vi "calib main.vi"() -> ()   [LabVIEW 2019]
uses:
  <vilib>/Utility/miscctls.llb/LVRowAndColumnTypeDef.ctl
  software/database.lvlib
  <vilib>/addons/Multicore Analysis and Sparse Matrix/Linear Algebra/NI_MASM_BasicLinAlg.lvlib
  <vilib>/Analysis/Matrix/NI_Matrix.lvlib
  software/detectedPellet.lvlib
  <vilib>/Analysis/Matrix/Numeric/Conversions/Array To Matrix - RA2.vi
  <vilib>/addons/Multicore Analysis and Sparse Matrix/Linear Algebra/_linalg/Solve Least Squares Problems (DBL).vi
panel:
  out "array":string[][](array[string])
  out "element":string
  out "Row":i32
  out "subarray":string[](array[string])
  out "Processing Table":string[][](table)
  in  "Numeric":i32=26
  in  "Stop (F)":bool
  out "Image Out":T1(plugin-control)
  out "output array":dbl[][](array[numeric])
  out "Error out":errorcluster
  in  "save_DB":bool
  out "Image":T1(plugin-control)
  in  "module path 2":path
  in  "process":bool
  out "Error out 5":errorcluster
  out "input array":dbl[][](array[numeric])
  out "known vector":dbl[](array[numeric])
  out "return value":dbl[](array[numeric])
  out "error out":errorcluster
  in  "module path":path
  out "Image Out 2":T1(plugin-control)
  out "Solution Vector":dbl[](array[numeric])
  in  "calculate":bool
  in  "capture":bool
  in  "snap number":u16(ring) items=["first", "second", "third"]
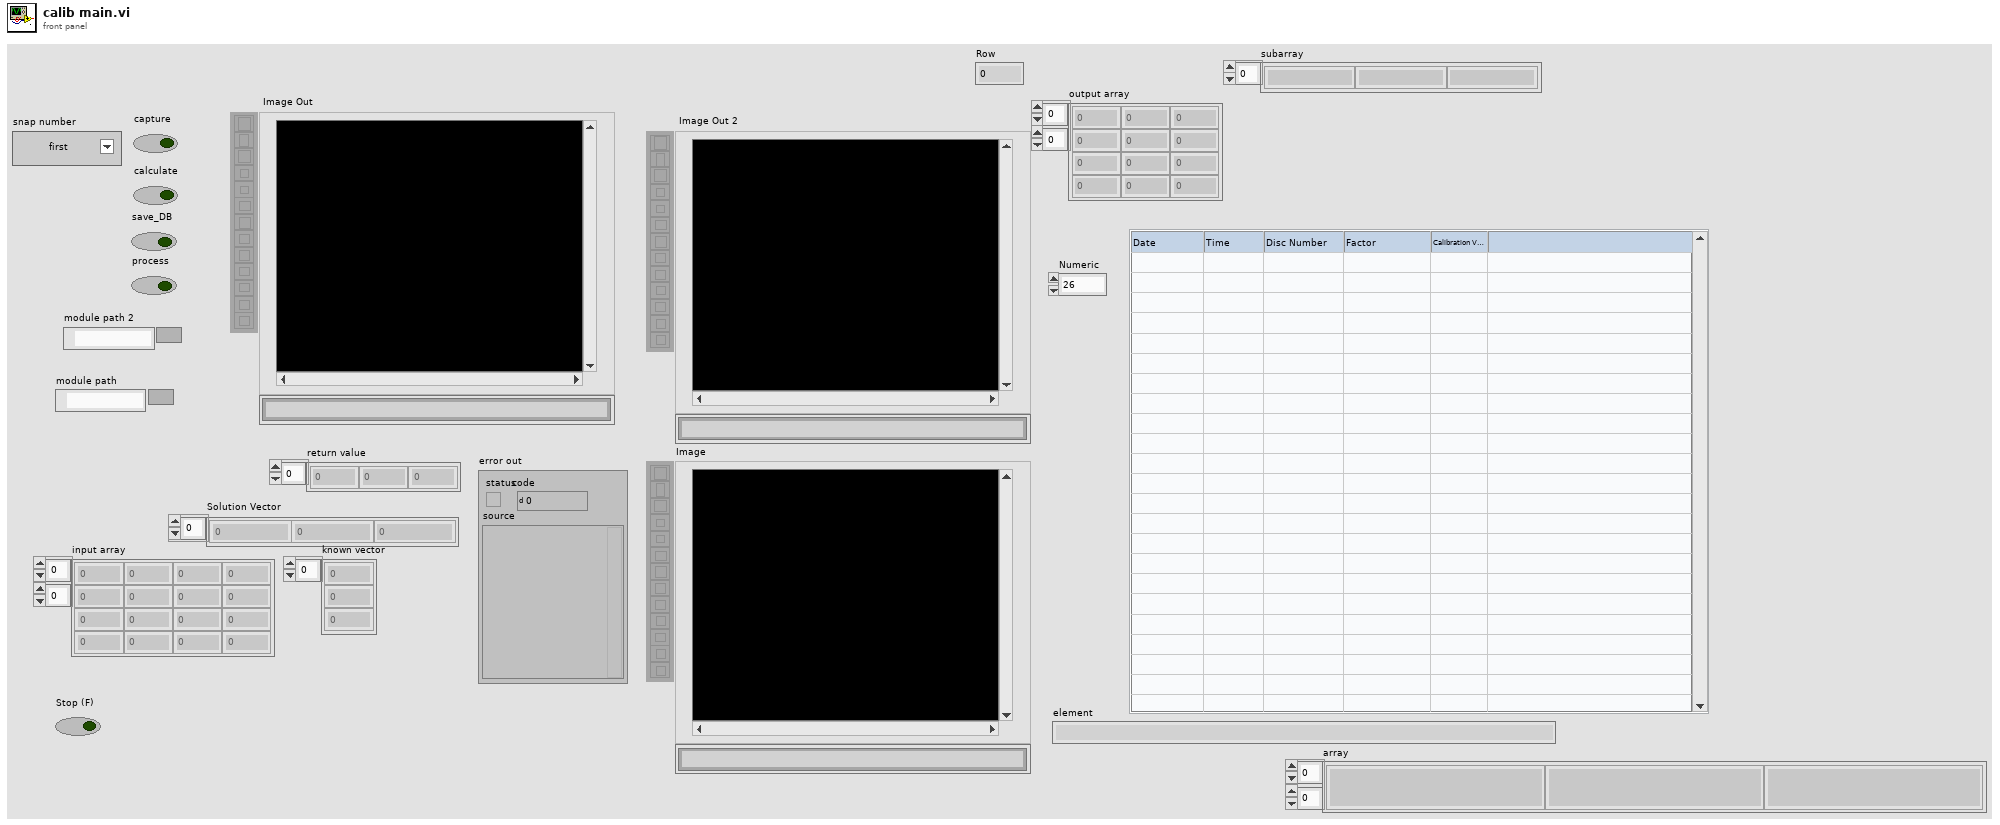
[diagram p1: front panel]
types:
  T1 = typedef "IMAQ Image.ctl" = refnum<image>
  T2 = typedef "Image Type" = u32
  T3 = typedef "LVRowAndColumnTypeDef.ctl" = cluster{"Row":i32, "Column":i32}
  T4 = cluster{"date/time string":string, "date/time string":string, "Numeric":i32, "spreadsheet string":string, "spreadsheet string":string}
  T5 = typedef "NI_Matrix.lvlib/RealMatrix.ctl" = dbl[][]
  T6 = cluster{"date/time string":string, "date/time string":string, "Numeric":dbl, "Numeric":dbl, "Numeric":dbl}
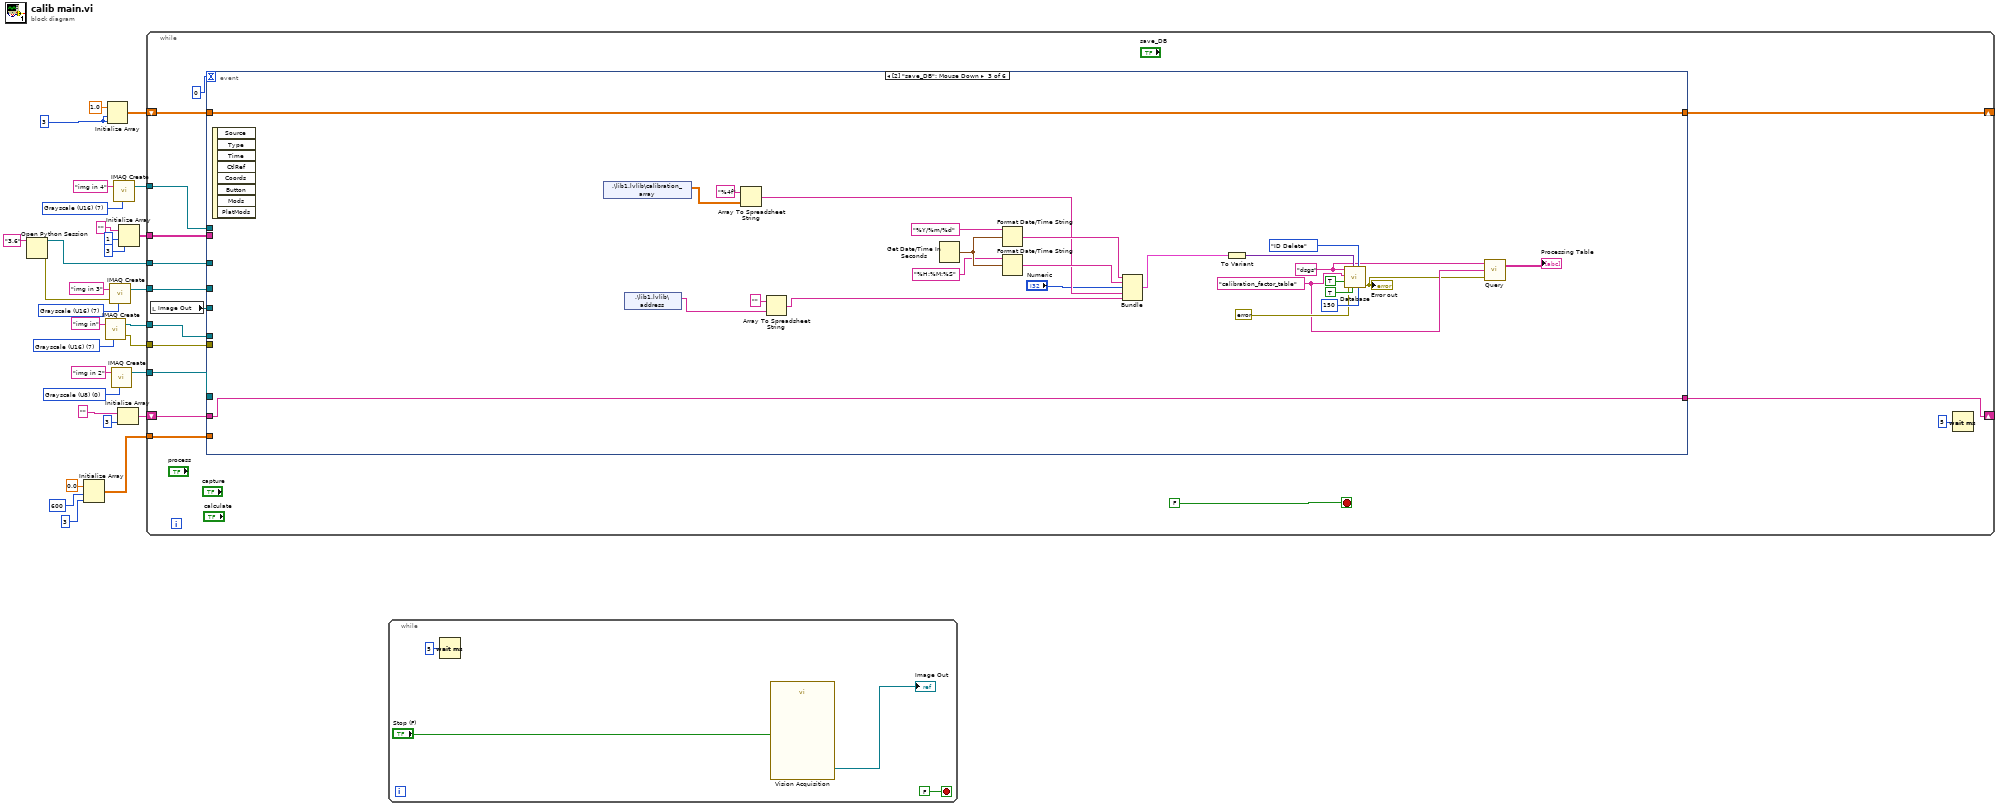
[diagram p0: block diagram]
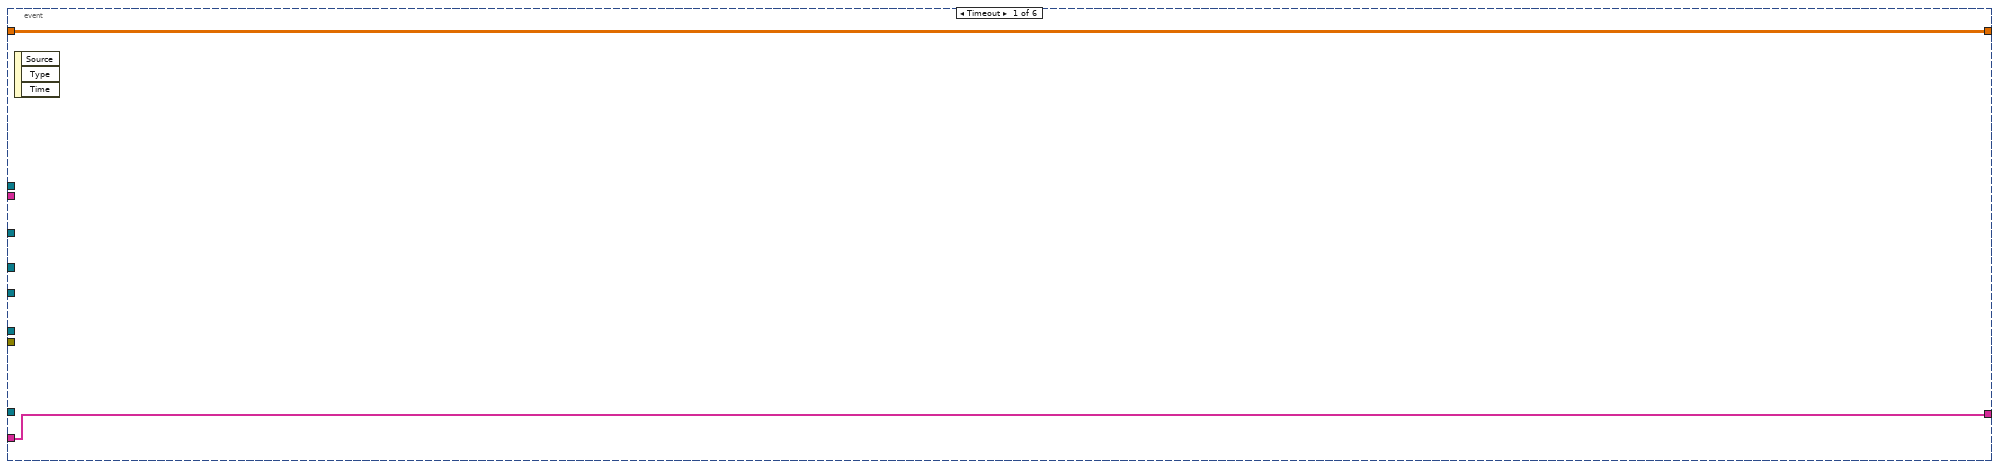
[diagram p2: hidden frame]
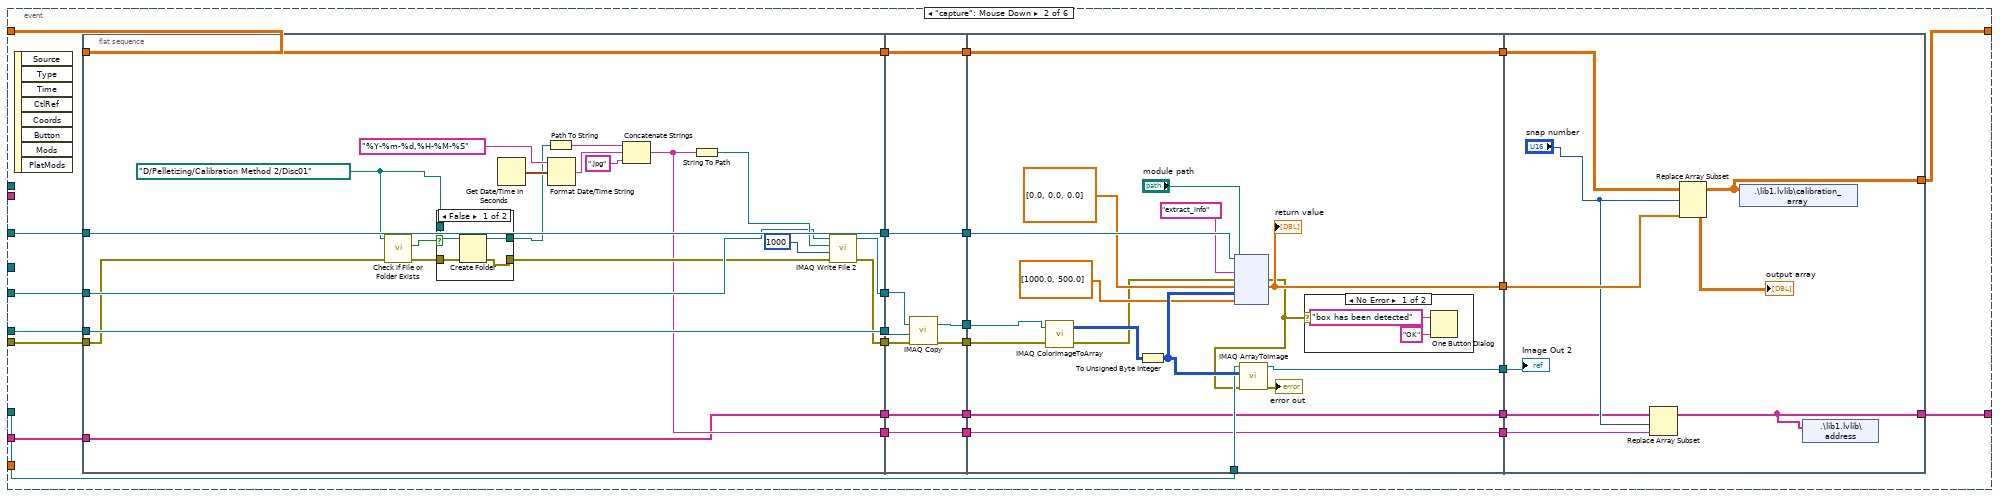
[diagram p3: hidden frame]
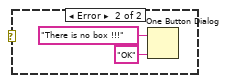
[diagram p5: hidden frame]
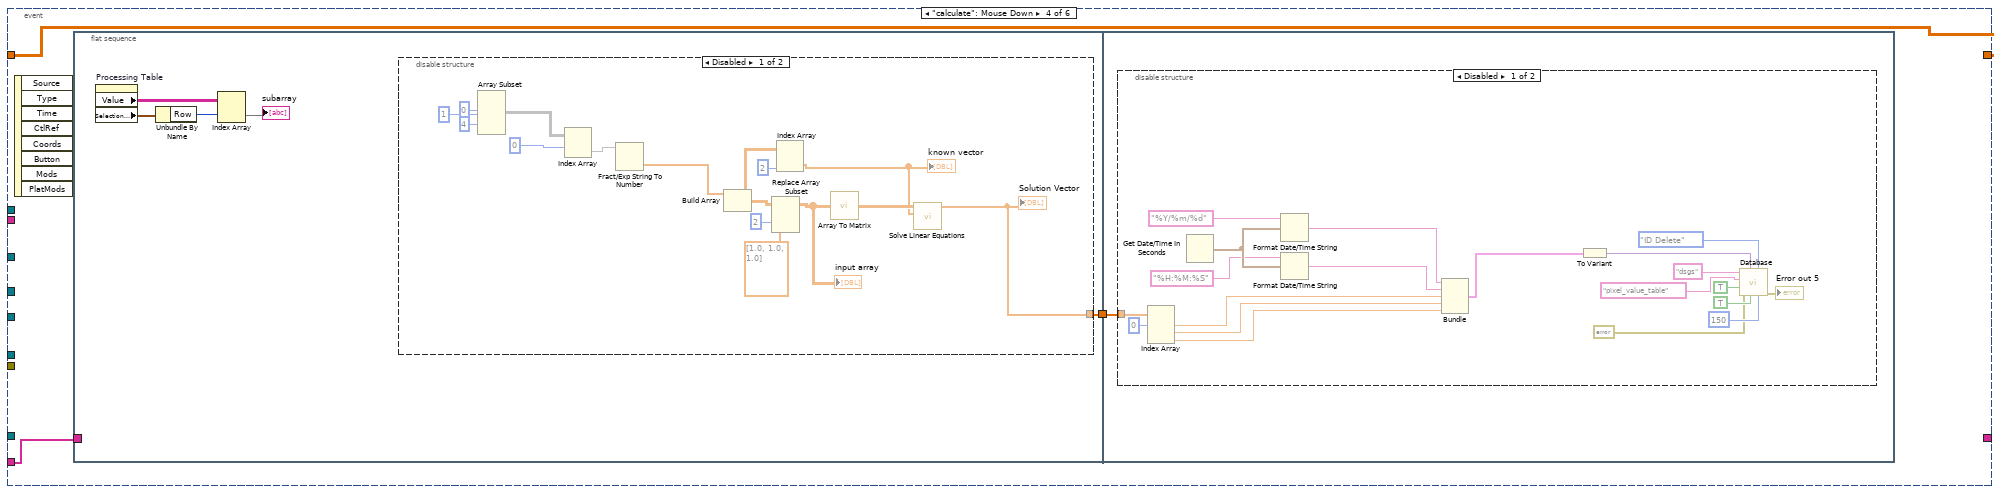
[diagram p6: hidden frame]
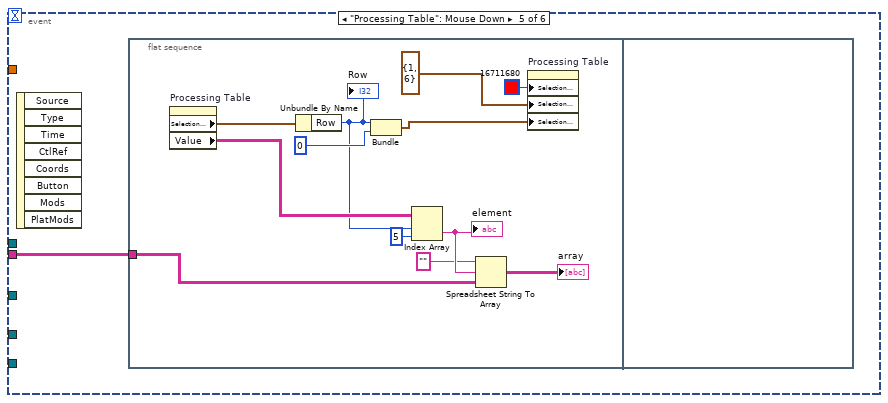
[diagram p9: hidden frame]
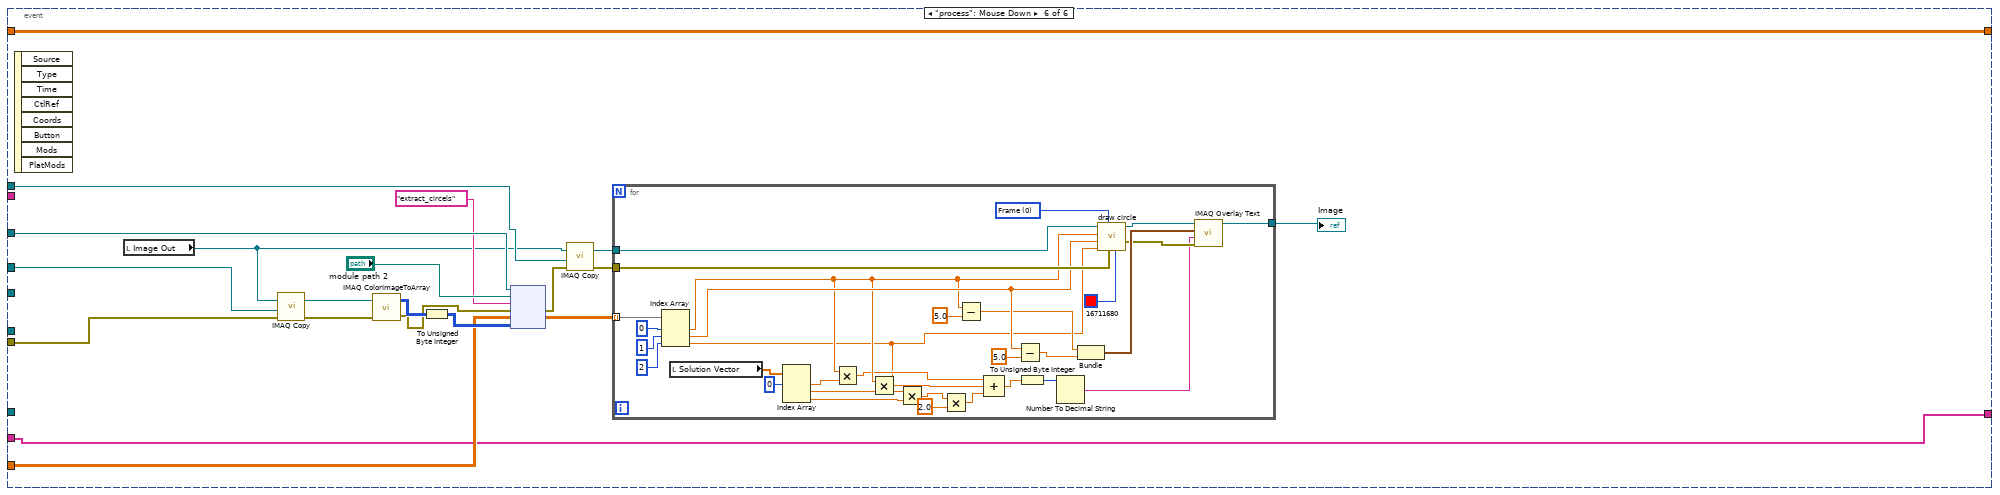
[diagram p10: hidden frame]
diagram:
  w9 = 3 ("dimension size")
  w12 = T2 7 items=["Grayscale (U8)", "Grayscale (I16)", "Grayscale (SGL)", "Complex (CSG)", "RGB (U32)", "HSL (U32)", "RGB (U64)", "Grayscale (U16)"] ("Image Type")
  w21 = T2 7 items=["Grayscale (U8)", "Grayscale (I16)", "Grayscale (SGL)", "Complex (CSG)", "RGB (U32)", "HSL (U32)", "RGB (U64)", "Grayscale (U16)"] ("Image Type")
  w24 = T2 0 items=["Grayscale (U8)", "Grayscale (I16)", "Grayscale (SGL)", "Complex (CSG)", "RGB (U32)", "HSL (U32)", "RGB (U64)", "Grayscale (U16)"] ("Image Type")
  w26 = T2 7 items=["Grayscale (U8)", "Grayscale (I16)", "Grayscale (SGL)", "Complex (CSG)", "RGB (U32)", "HSL (U32)", "RGB (U64)", "Grayscale (U16)"] ("Image Type")
  n1 = Open Python Session(python version="3.6" ("Python version")) -> (session out=w29:refnum<k35>, error out=w19:errorcluster)  [unwired: 2 in]
  n2 = Initialize Array(0.0 ("element"), 600 ("dimension size"), 3 ("dimension size")) -> (w14:dbl[][])
  n3 = call "IMAQ Create"("Image Name"="img in", "Image Type"=w26) -> ("New Image"=w27:T1, "error out"=w25:errorcluster)  [unwired: 3 in]
  n4 = Initialize Array(1.0 ("element"), w9, w9) -> (w8:dbl[][])
  n5 = call "IMAQ Create"("Image Name"="img in 3", "Image Type"=w21, "error in (no error)"=w19) -> ("New Image"=w18:T1)  [unwired: 2 in, 1 out]
  n6 = call "IMAQ Create"("Image Name"="img in 2", "Image Type"=w24) -> ("New Image"=w22:T1)  [unwired: 3 in, 1 out]
  n7 = call "IMAQ Create"("Image Name"="img in 4", "Image Type"=w12) -> ("New Image"=w11:T1)  [unwired: 3 in, 1 out]
  n8 = Initialize Array("", 3 ("dimension size")) -> (w5:string[])
  n9 = Initialize Array("", 1 ("dimension size"), 3 ("dimension size")) -> (w1:string[][])
  n10 = while {
    tunnel: w29 -> [w43]
    tunnel: w27 -> [w42]
    tunnel: w25 -> [w41]
    tunnel: w22 -> [w40]
    tunnel: w18 -> [w39]
    tunnel: w14 -> [w38]
    tunnel: w11 -> [w37]
    shift-right: [w35] -> _
    shift-left: w8 -> [w36]
    shift-right: [w32] -> _
    shift-left: w5 -> [w33]
    tunnel: w1 -> [w31]
    stop <- FALSE stop-if-true
    n11 = local read "Image Out"() -> (w34:T1)
    n12 = event shown="[2] \"save_DB\": Mouse Down" {
      selector: _ -> [_ _ _ _ _ _]
      dyn-events: _ -> [_ _ _ _ _ _]
      timeout: 0 -> [_ _ _ _ _ _]
      tunnel: w43 -> [_ w75 _ _ _ w239]
      tunnel: w42 -> [_ w73 _ _ _ _]
      tunnel: w41 -> [_ w70 _ _ _ w242]
      tunnel: w40 -> [_ w69 _ _ _ _]
      tunnel: w39 -> [_ _ _ _ _ w243]
      tunnel: w38 -> [_ _ _ _ _ w234]
      tunnel: w37 -> [_ _ _ _ _ w228]
      tunnel: w36 -> [w48 w66 w150 w168 _ w225]
      tunnel: [w48 w63 w150 w168 _ w225] -> w35
      tunnel: w34 -> [_ w62 _ _ _ _]
      tunnel: w33 -> [w47 w50 w149 w167 _ w224]
      tunnel: [w47 w49 w149 _ _ w224] -> w32
      tunnel: w31 -> [_ _ _ _ w211 _]
      event Timeout {
        n13 = event-data() -> ()  [unwired: 1 in, 3 out]
      }
      event "capture": Mouse Down {
        n14 = event-data() -> ()  [unwired: 1 in, 8 out]
        n15 = flat-sequence {
          tunnel: w62 -> [w86]
          tunnel: w66 -> [w94]
          tunnel: w70 -> [w85]
          tunnel: w73 -> [w95]
          tunnel: w75 -> [w96]
          tunnel: [w96] -> w61
          tunnel: [w95] -> w60
          tunnel: [w83] -> w59
          tunnel: [w94] -> w58
          tunnel: [w78] -> w57
          tunnel: [w77] -> w54
          tunnel: [w76] -> w51
          tunnel: w50 -> [w76]
          tunnel: [w111] -> w74
          tunnel: [w109] -> w72
          tunnel: [w108] -> w71
          tunnel: [w106] -> w65
          tunnel: w61 -> [w111]
          tunnel: w60 -> [w110]
          tunnel: w59 -> [w107]
          tunnel: w58 -> [w106]
          tunnel: w57 -> [w105]
          tunnel: [w104] -> w55
          tunnel: w54 -> [w104]
          tunnel: [w103] -> w52
          tunnel: w51 -> [w103]
          tunnel: w74 -> [w126]
          tunnel: w72 -> [w129]
          tunnel: w71 -> [w128]
          tunnel: w69 -> [w124]
          tunnel: [w123] -> w67
          tunnel: [w117] -> w68
          tunnel: w65 -> [w116]
          tunnel: [w116] -> w64
          tunnel: [w113] -> w56
          tunnel: w55 -> [w113]
          tunnel: [w112] -> w53
          tunnel: w52 -> [w112]
          tunnel: w64 -> [w140]
          tunnel: w67 -> [w141]
          tunnel: w68 -> [w138]
          tunnel: [w139] -> w63
          tunnel: w56 -> [w137]
          tunnel: w53 -> [w135]
          tunnel: [w134] -> w49
          frame #0 {
            w81 = path "D:/Pelletizing/Calibration Method 2/Disc01" ("path")
            n16 = call <vilib>:"Check if File or Folder Exists.vi"("error in (no error)"=w85, "path"=w81) -> ("error out"=w84:errorcluster, "file or folder exists?"=w82:bool)  [unwired: 7 in, 1 out]
            n17 = case shown="False" w82 {
              tunnel: w84 -> [w100 w102]
              tunnel: [w99 w102] -> w80
              tunnel: w81 -> [w98 w101]
              tunnel: [w97 w101] -> w79
              frame False {
                n18 = Create Folder(path (use dialog)=w98, error in=w100) -> (created path=w97:path, error out=w99:errorcluster)  [unwired: 1 in, 1 out]
              }
              frame True {
              }
            }
            n19 = Get Date/Time In Seconds() -> (seconds since 1Jan1904=w92:timestamp)
            n20 = Path To String(path=w79) -> (string=w87:string)
            n21 = Format Date/Time String(time format string (%c)="%Y-%m-%d,%H-%M-%S", seconds (now)=w92) -> (date/time string=w90:string)  [unwired: 1 in]
            n22 = Concatenate Strings(w87, w90, ".jpg" ("string")) -> (w77:string)
            n23 = String To Path(string=w77) -> (path=w88:path)
            n24 = call-poly "IMAQ Write File 2"("error in (no error)"=w80, "Image Quality"=u32 1000, "File Path"=w88, "Image"=w86) -> ("error out"=w83:errorcluster, "Image Out (duplicate)"=w78:T1)  [unwired: 6 in]
          }
          frame #1 {
            n25 = call "IMAQ Copy"("error in (no error)"=w107, "Image Dst"=w110, "Image Src"=w105) -> ("error out"=w108:errorcluster, "Image Dst Out"=w109:T1)  [unwired: 3 in]
          }
          frame #2 {
            n26 = call "IMAQ ColorImageToArray"("Image"=w129, "error in (no error)"=w128) -> ("Image Pixels (U32)"=w127:u32[][], "error out"=w115:errorcluster)  [unwired: 2 in, 1 out]
            n27 = To Unsigned Byte Integer(number=w127) -> (unsigned 8bit integer=w125:u8[][])
            n28 = node(w126, "module path", "extract_info" ("function name"), w115, dbl[] [0.0, 0.0, 0.0], w125, dbl[] [1000.0, 500.0]) -> (w114:errorcluster, w117:dbl[])  [unwired: 2 in, 3 out]
            "return value" <- w117
            n29 = call "IMAQ ArrayToImage"("error in (no error)"=w114, "Image Pixels (U8)"=w125, "Image"=w124) -> ("error out"=→"error out":errorcluster, "Image Out"=w123:T1)  [unwired: 7 in]
            n30 = case shown="No Error" w114 {
              frame No Error {
                n31 = One Button Dialog(message="box has been detected", button name ("OK")="OK") -> ()  [unwired: 1 out]
              }
              frame Error {
                n32 = One Button Dialog(message="There is no box !!!", button name ("OK")="OK") -> ()  [unwired: 1 out]
              }
            }
          }
          frame #3 {
            n33 = Replace Array Subset(array=w135, new element=w137, index="snap number") -> (w134:string[])
            n34 = Replace Array Subset(array=w140, new element=w138, index (row)="snap number") -> (w139:dbl[][])  [unwired: 1 in]
            "output array" <- w139
            n35 = shared-variable ".\\lib1.lvlib\\calibration_array"(w139) -> ()  [unwired: 1 in, 1 out]
            n36 = shared-variable ".\\lib1.lvlib\\address"(w134) -> ()  [unwired: 1 in, 1 out]
            "Image Out 2" <- w141
          }
        }
      }
      event "save_DB": Mouse Down {
        w147 = "calibration_factor_table" ("Table")
        w148 = "dsgs" ("Connection")
        n37 = event-data() -> ()  [unwired: 1 in, 8 out]
        n38 = shared-variable ".\\lib1.lvlib\\calibration_array"() -> (w154:dbl[][])  [unwired: 1 in, 1 out]
        n39 = shared-variable ".\\lib1.lvlib\\address"() -> (w144:string[])  [unwired: 1 in, 1 out]
        n40 = Array To Spreadsheet String(array=w154, 3:"%4f" ("format string")) -> (spreadsheet string=w152:string)  [unwired: 1 in]
        n41 = Array To Spreadsheet String(array=w144, 3:"" ("format string")) -> (spreadsheet string=w142:string)  [unwired: 1 in]
        n42 = Get Date/Time In Seconds() -> (seconds since 1Jan1904=w158:timestamp)
        n43 = Format Date/Time String(time format string (%c)="%Y/%m/%d", seconds (now)=w158) -> (date/time string=w159:string)  [unwired: 1 in]
        n44 = Format Date/Time String(time format string (%c)="%H:%M:%S", seconds (now)=w158) -> (date/time string=w157:string)  [unwired: 1 in]
        n45 = Bundle("date/time string"=w159, "date/time string"=w157, "Numeric"="Numeric", "spreadsheet string"=w152, "spreadsheet string"=w142) -> (w161:T4)  [unwired: 1 in]
        n46 = To Variant(anything=w161) -> (Variant=w166:variant)
        n47 = call "Database.vi"("Maximum Row"=150, "Enum"=enum16{"ID Delete", "Time Delete"}."ID Delete", "Delete row?"=TRUE, "Data"=w166, "Error in"=errorcluster {"status"=FALSE, "code"=0, "source"=""}, "Auto Increment ID?"=TRUE, "Table"=w147, "Connection"=w148) -> ("Error out"=w146:errorcluster)  [unwired: 3 in]
        "Error out" <- w146
        n48 = call "Query.vi"("Error in"=w146, "Table Name"=w147, "Connection Name"=w148) -> ("data"=→"Processing Table":string[][])  [unwired: 1 in, 1 out]
      }
      event "calculate": Mouse Down {
        n49 = event-data() -> ()  [unwired: 1 in, 8 out]
        n50 = flat-sequence {
          tunnel: [w174] -> w169
          tunnel: w167 -> [_]
          tunnel: w169 -> [w190]
          frame #0 {
            n51 = property on="Processing Table" class="Tbl (strict)"() -> ("Value"=w173:string[][], "Selection Start"=w172:T3)  [unwired: 2 in, 2 out]
            n52 = Unbundle By Name(w172) -> ("Row"=w171:i32)
            n53 = Index Array(array=w173, index (row)=w171) -> (element=→"subarray":string[])  [unwired: 1 in]
            n54 = disable-structure shown="Disabled" {
              disable-tunnel: [w175 _] -> w174
              frame Disabled {
                n55 = Array Subset(index (row)=0 ("index"), length (row)=1 ("length"), index (col)=4 ("index")) -> (w186:void[][])  [unwired: 2 in]
                n56 = Index Array(array=w186, index (row)=0 ("disabled index (row)")) -> (element=w185:void[])  [unwired: 1 in]
                n57 = Fract/Exp String To Number(string=w185) -> (number=w183:dbl[])  [unwired: 3 in, 1 out]
                n58 = Build Array(w183) -> (w179:dbl[][])  [unwired: 2 in]
                n59 = Replace Array Subset(array=w179, new element=dbl[] [1.0, 1.0, 1.0] ("new element/subarray"), index (col)=2 ("disabled index (col)")) -> (w176:dbl[][])  [unwired: 1 in]
                "input array" <- w176
                n60 = Index Array(array=w179, index (col)=2 ("disabled index (col)")) -> (element=w177:dbl[])  [unwired: 1 in]
                "known vector" <- w177
                n61 = call-poly <vilib>:"Array To Matrix.vi"("Real 2D Array"=w176) -> ("Real Matrix"=w182:T5)
                n62 = call-poly <vilib>:"Solve Linear Equations.vi"("Known Vector"=w177, "Input Matrix"=w182) -> ("Solution Vector"=w175:dbl[])  [unwired: 8 in, 1 out]
                "Solution Vector" <- w175
              }
              frame Enabled {
              }
            }
          }
          frame #1 {
            n63 = disable-structure shown="Disabled" {
              disable-tunnel: w190 -> [w196 _]
              frame Disabled {
                n64 = Index Array(array=w196, index #1=0 ("index")) -> (element #1=w194:dbl, element #2=w193:dbl, element #3=w192:dbl)  [unwired: 2 in]
                n65 = Get Date/Time In Seconds() -> (seconds since 1Jan1904=w209:timestamp)
                n66 = Format Date/Time String(time format string (%c)="%Y/%m/%d", seconds (now)=w209) -> (date/time string=w210:string)  [unwired: 1 in]
                n67 = Format Date/Time String(time format string (%c)="%H:%M:%S", seconds (now)=w209) -> (date/time string=w208:string)  [unwired: 1 in]
                n68 = Bundle("date/time string"=w210, "date/time string"=w208, "Numeric"=w194, "Numeric"=w193, "Numeric"=w192) -> (w191:T6)  [unwired: 1 in]
                n69 = To Variant(anything=w191) -> (Variant=w205:variant)
                n70 = call "Database.vi"("Maximum Row"=150, "Enum"=enum16{"ID Delete", "Time Delete"}."ID Delete", "Delete row?"=TRUE, "Data"=w205, "Error in"=errorcluster {"status"=FALSE, "code"=0, "source"=""}, "Auto Increment ID?"=TRUE, "Table"="pixel_value_table", "Connection"="dsgs") -> ("Error out"=→"Error out 5":errorcluster)  [unwired: 3 in]
              }
              frame Enabled {
              }
            }
          }
        }
      }
      event "Processing Table": Mouse Down {
        n71 = event-data() -> ()  [unwired: 1 in, 8 out]
        n72 = flat-sequence {
          tunnel: w211 -> [w214]
          frame #0 {
            n73 = property on="Processing Table" class="Tbl (strict)"() -> ("Selection Start"=w222:T3, "Value"=w218:string[][])  [unwired: 2 in, 2 out]
            n74 = Unbundle By Name(w222) -> ("Row"=w217:i32)
            "Row" <- w217
            n75 = Bundle("Row"=w217, 0) -> (w220:cluster{"Row":i32, i32})  [unwired: 1 in]
            n76 = Index Array(array=w218, index (row)=w217, index (col)=5 ("disabled index (col)")) -> (element=w215:string)
            "element" <- w215
            n77 = Spreadsheet String To Array(format string="", spreadsheet string=w215, array type (2D Dbl)=w214) -> (array=→"array":string[][])  [unwired: 1 in]
            n78 = property on="Processing Table" class="Tbl (strict)"("Selection Color"=u32 16711680, "Selection Size"=T3 {"Row"=1, "Column"=6}, "Selection Start"=w220) -> ()  [unwired: 2 in, 2 out]
          }
          frame #1 {
          }
        }
      }
      event "process": Mouse Down {
        n79 = event-data() -> ()  [unwired: 1 in, 8 out]
        n80 = local read "Image Out"() -> (w227:T1)
        n81 = call "IMAQ Copy"("error in (no error)"=w242, "Image Dst"=w243, "Image Src"=w227) -> ("error out"=w240:errorcluster, "Image Dst Out"=w241:T1)  [unwired: 3 in]
        n82 = call "IMAQ ColorImageToArray"("Image"=w241, "error in (no error)"=w240) -> ("Image Pixels (U32)"=w236:u32[][], "error out"=w231:errorcluster)  [unwired: 2 in, 1 out]
        n83 = To Unsigned Byte Integer(number=w236) -> (unsigned 8bit integer=w235:u8[][])
        n84 = node(w239, "module path 2", "extract_circels" ("function name"), w231, w234, w235) -> (w230:errorcluster, w233:dbl[][])  [unwired: 1 in, 3 out]
        n85 = call "IMAQ Copy"("error in (no error)"=w230, "Image Dst"=w228, "Image Src"=w227) -> ("error out"=w229:errorcluster, "Image Dst Out"=w232:T1)  [unwired: 3 in]
        n86 = for {
          tunnel: w232 -> [w275]
          tunnel: w233 -> [w274] mode=indexing
          tunnel: w229 -> [w269]
          tunnel: [w257] -> w226
          w270 = u32 0 items=["Frame", "Fill"] ("Drawing Mode (Frame)")
          n87 = Index Array(array=w274, index #1=0 ("index"), index #2=1 ("index"), index #3=2 ("index")) -> (element #1=w252:dbl, element #2=w265:dbl, element #3=w248:dbl)
          n88 = local read "Solution Vector"() -> (w256:dbl[])
          n89 = Index Array(array=w256, index #1=0 ("index")) -> (element #1=w254:dbl, element #2=w253:dbl, element #3=w247:dbl)  [unwired: 2 in]
          n90 = Multiply(x=w252, y=w254) -> (x*y=w251:dbl)
          n91 = Multiply(x=w252, y=w253) -> (x*y=w249:dbl)
          n92 = Multiply(x=w248, y=w247) -> (x*y=w246:dbl)
          n93 = Multiply(x=w246, y=2.0) -> (x*y=w244:dbl)
          n94 = Subtract(x=w252, y=5.0) -> (x-y=w264:dbl)
          n95 = Compound Arithmetic op=ADD(w251, w249, w244) -> (w250:dbl)
          n96 = Subtract(x=w265, y=5.0) -> (x-y=w263:dbl)
          n97 = To Unsigned Byte Integer(number=w250) -> (unsigned 8bit integer=w260:u8)
          n98 = Number To Decimal String(number=w260) -> (decimal integer string=w259:string)  [unwired: 1 in]
          n99 = Bundle(w264, w263) -> (w262:cluster{dbl, dbl})  [unwired: 1 in]
          n100 = call "draw circle.vi"("Color"=u32 16711680, "error in (no error)"=w269, "Drawing Mode (Frame)"=w270, "box size"=w248, "Y"=w265, "X"=w252, "Image In"=w275) -> ("error out"=w261:errorcluster, "Image Out"=w258:T1)  [unwired: 3 in]
          n101 = call "IMAQ Overlay Text"("error in (no error)"=w261, "String"=w259, "Origin"=w262, "Image"=w258) -> ("Image Out"=w257:T1)  [unwired: 6 in, 1 out]
        }
        "Image" <- w226
      }
    }
    n102 = Wait (ms)(milliseconds to wait=u32 5) -> ()  [unwired: 1 out]
  }
  n103 = while {
    stop <- FALSE stop-if-true
    n104 = Wait (ms)(milliseconds to wait=u32 5) -> ()  [unwired: 1 out]
    n105 = call "Vision Acquisition"("Stop (F)"="Stop (F)") -> ("Image Out"=→"Image Out":T1)  [unwired: 24 in, 2 out]
  }
